vi "Do Open Vi.vi"(8 "error in (no error)":errorcluster, 10 "open_vi Argument":T4, 11 "Data Cluster in":T1) -> (0 "error out":errorcluster, 2 "open_vi (Reply Payload)":T3, 3 "Data Cluster out":T1)   [LabVIEW 2025, in "Scripting Server.lvlib"]
uses:
  Scripting Server.lvlib
  open_vi (Reply Payload)--cluster.ctl
  open_vi Argument--cluster.ctl
  Config Data.ctl
  Module Data--cluster.ctl
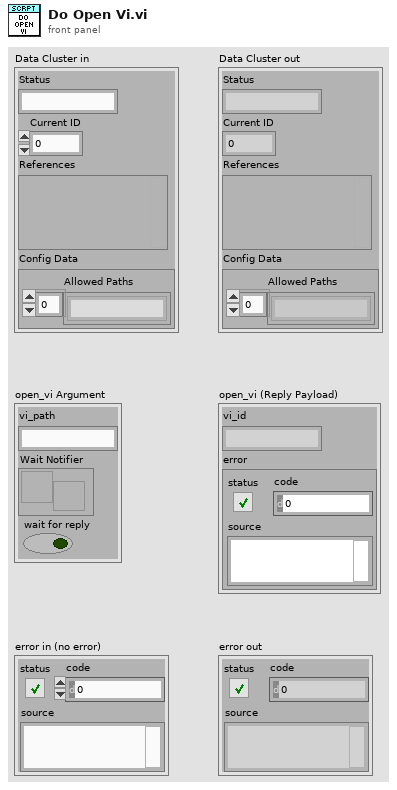
[diagram p1: front panel]
types:
  T1 = typedef "Scripting Server.lvlib/Module Data--cluster.ctl" = cluster{"Status":string, "Current ID":i32, "References":variant, "Config Data":T2}
  T2 = typedef "Scripting Server.lvlib/Config Data.ctl" = cluster{"Allowed Paths":string[]}
  T3 = typedef "Scripting Server.lvlib/open_vi (Reply Payload)--cluster.ctl" = cluster{"vi_id":string, "error":errorcluster}
  T4 = typedef "Scripting Server.lvlib/open_vi Argument--cluster.ctl" = cluster{"vi_path":string, "Wait Notifier":refnum<notifier>, "wait for reply":bool}
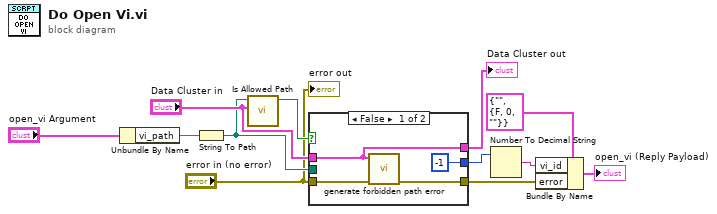
[diagram p0: block diagram]
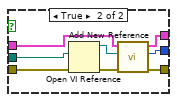
[diagram p2: hidden frame]
diagram:
  n1 = Unbundle By Name("open_vi Argument") -> ("vi_path"=w7:string)
  n2 = String To Path(string=w7) -> (path=w5:path)
  n3 = call "Is Allowed Path.vi"("Data Cluster in"="Data Cluster in", "Path"=w5) -> ("Forbidden"=w6:bool)  [unwired: 9 in]
  n4 = case shown="False" w6 {
    tunnel: "error in (no error)" -> [w16 w24]
    tunnel: [w15 w23] -> w2
    tunnel: "Data Cluster in" -> [w14 w22]
    tunnel: [w14 w21] -> w9
    tunnel: w5 -> [_ w19]
    tunnel: [-1 ("new reference") w17] -> w4
    frame False {
      n5 = call "generate forbidden path error.vi"("error in (no error)"=w16, "Data Cluster in"=w14) -> ("error out"=w15:errorcluster)  [unwired: 9 in]
    }
    frame True {
      n6 = Open VI Reference(vi path=w19, error in (no error)=w24) -> (vi reference=w18:refnum<vi>, error out=w20:errorcluster)  [unwired: 4 in]
      n7 = call "Add New Reference.vi"("error in (no error)"=w20, "Variant"=w18, "Data Cluster in"=w22) -> ("error out"=w23:errorcluster, "new reference"=w17:i32, "Data Cluster out 2"=w21:T1)  [unwired: 6 in]
    }
  }
  "Data Cluster out" <- w9
  n8 = Number To Decimal String(number=w4) -> (decimal integer string=w3:string)  [unwired: 1 in]
  n9 = Bundle By Name(cluster=T3 {"vi_id"="", "error"={"status"=FALSE, "code"=0, "source"=""}} ("open_vi (Reply Payload)"), "vi_id"=w3, "error"=w2) -> (→"open_vi (Reply Payload)":T3)
  "error out" <- "error in (no error)"
